vi "Set Output Values.vi"(8 "error in (no error)":errorcluster, 11 "Spectrum Recorder in":refnum<class "Spectrum Recorder.lvclass">) -> (0 "error out":errorcluster, 3 "Spectrum Recorder out":refnum<class "Spectrum Recorder.lvclass">)   [LabVIEW 2016, in "Spectrum Recorder.lvclass"]
uses:
  Spectrum Recorder.lvclass
  Spectrum Recorder.lvclass/Spectrum Recorder.ctl
  Red Pitaya/RP Core/RP Transceiver/RP Transceiver.lvclass
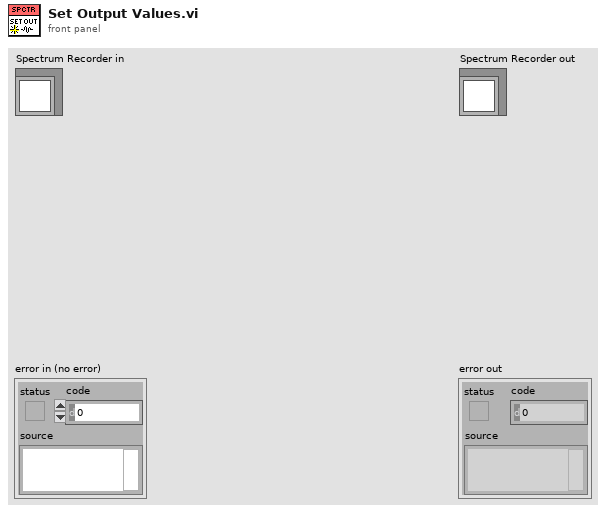
[diagram p1: front panel]
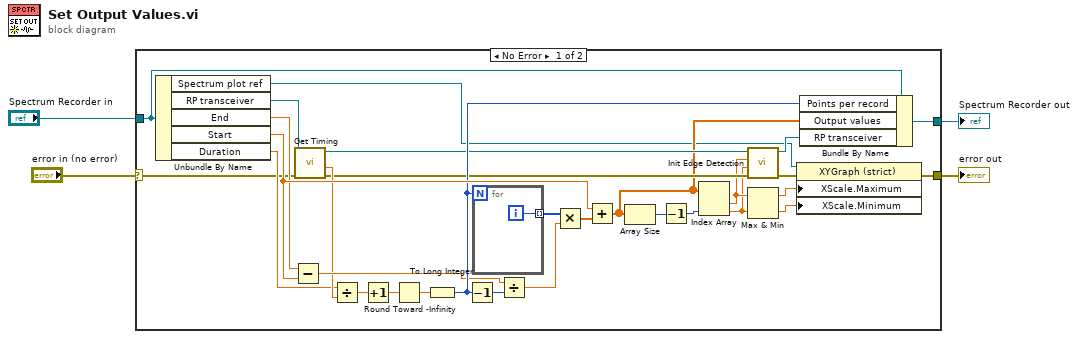
[diagram p0: block diagram]
diagram:
  n1 = case shown="No Error" "error in (no error)" {
    selector: "error in (no error)" -> [w19 w37]
    tunnel: [w11 w37] -> w3
    tunnel: [w21 w36] -> w1
    tunnel: "Spectrum Recorder in" -> [w20 w36]
    frame No Error {
      n2 = Unbundle By Name(w20) -> ("Spectrum plot ref"=w12:refnum<vi>, "RP transceiver"=w5:refnum<class "RP Transceiver.lvclass">, "End"=w22:dbl, "Start"=w33:dbl, "Duration"=w23:dbl)
      n3 = Subtract(x=w22, y=w33) -> (x-y=w29:dbl)
      n4 = call-dynamic "Get Timing.vi"("error in (no error)"=w19, "RP Transceiver in"=w5) -> ("error out"=w18:errorcluster, "dt"=w24:dbl, "RP Transceiver out"=w16:refnum<class "RP Transceiver.lvclass">)  [unwired: 5 in, 2 out]
      n5 = Divide(x=w23, y=w24) -> (x/y=w27:dbl)
      n6 = Increment(x=w27) -> (x+1=w26:dbl)
      n7 = Round Toward -Infinity(1:w26) -> (0:w25:dbl)
      n8 = To Long Integer(number=w25) -> (32bit integer=w30:i32)
      n9 = Decrement(x=w30) -> (x-1=w28:i32)
      n10 = for {
        N: w30 -> [_]
        tunnel: [w35] -> w32 mode=indexing
        i -> [w35]
      }
      n11 = Divide(x=w29, y=w28) -> (x/y=w31:dbl)
      n12 = Multiply(x=w32, y=w31) -> (x*y=w34:dbl[])
      n13 = Add(x=w33, y=w34) -> (x+y=w15:dbl[])
      n14 = Array Size(array=w15) -> (size(s)=w14:i32)
      n15 = Decrement(x=w14) -> (x-1=w13:i32)
      n16 = Index Array(array=w15, index #2=w13) -> (element #1=w9:dbl, element #2=w8:dbl)  [unwired: 1 in]
      n17 = call-dynamic "Init Edge Detection.vi"("error in (no error)"=w18, "Last output"=w8, "First output"=w9, "RP Transceiver in"=w16) -> ("error out"=w10:errorcluster, "RP Transceiver out"=w17:refnum<class "RP Transceiver.lvclass">)  [unwired: 6 in]
      n18 = Max & Min(x=w9, y=w8) -> (max(x,y)=w7:dbl, min(x,y)=w6:dbl)
      n19 = property class="XYGraph (strict)"(reference=w12, error in=w10, "XScale.Maximum"=w7, "XScale.Minimum"=w6) -> (error out=w11:errorcluster)  [unwired: 1 out]
      n20 = Bundle By Name(cluster=w20, "Points per record"=w30, "Output values"=w15, "RP transceiver"=w17) -> (w21:refnum<class "Spectrum Recorder.lvclass">)
    }
    frame Error {
    }
  }
  "error out" <- w3
  "Spectrum Recorder out" <- w1
